vi "Convert a number to its letter.vi"(2 "Number":i32, 3 "ordered item type (default)":T1(ring)) -> (1 "string":string)   [LabVIEW 2015, in "NI_ReportGenerationCore.lvlib"]
uses:
  <vilib>/Utility/NIReport.llb/NI_ReportGenerationCore.lvlib
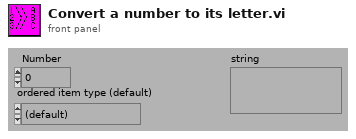
[diagram p1: front panel]
types:
  T1 = enum16{"(default)", "arabic numerals", "lower alpha", "upper alpha"}
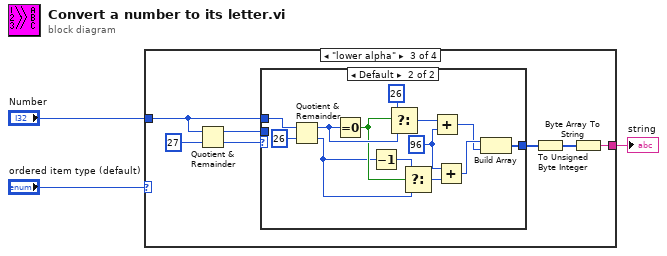
[diagram p0: block diagram]
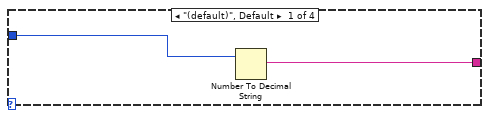
[diagram p2: hidden frame]
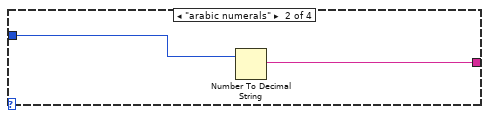
[diagram p3: hidden frame]
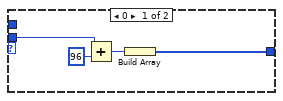
[diagram p4: hidden frame]
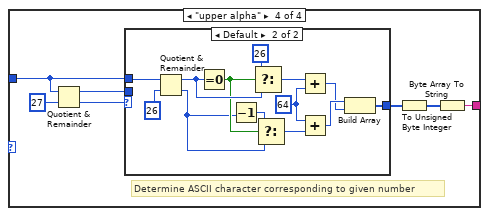
[diagram p5: hidden frame]
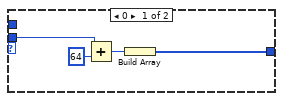
[diagram p6: hidden frame]
diagram:
  n1 = case shown="\"lower alpha\"" "ordered item type (default)" {
    tunnel: [w5 w7 w10 w34] -> w3
    tunnel: "Number" -> [w4 w6 w9 w33]
    frame "(default)", Default {
      n2 = Number To Decimal String(number=w4) -> (decimal integer string=w5:string)  [unwired: 1 out]
    }
    frame "arabic numerals" {
      n3 = Number To Decimal String(number=w6) -> (decimal integer string=w7:string)  [unwired: 1 out]
    }
    frame "lower alpha" {
      n4 = Quotient & Remainder(x=w9, y=27) -> (x-y*floor(x/y)=w13:i32, floor(x/y)=w8:i32)
      n5 = case shown="Default" w8 {
        tunnel: w9 -> [_ w19]
        tunnel: w13 -> [w18 _]
        tunnel: [w17 w21] -> w12
        frame 0 {
          n6 = Add(x=w18, y=96) -> (x+y=w15:i32)
          n7 = Build Array(w15) -> (w17:i32[])
        }
        frame Default {
          w20 = 96
          n8 = Quotient & Remainder(x=w19, y=26) -> (x-y*floor(x/y)=w29:i32, floor(x/y)=w26:i32)
          n9 = Equal To 0?(x=w29) -> (x = 0?=w27:bool)
          n10 = Decrement(x=w26) -> (x-1=w28:i32)
          n11 = Select(t=26, s=w27, f=w29) -> (s? t:f=w25:i32)
          n12 = Select(t=w28, s=w27, f=w26) -> (s? t:f=w24:i32)
          n13 = Add(x=w25, y=w20) -> (x+y=w22:i32)
          n14 = Add(x=w20, y=w24) -> (x+y=w23:i32)
          n15 = Build Array(w23, w22) -> (w21:i32[])
        }
      }
      n16 = To Unsigned Byte Integer(number=w12) -> (unsigned 8bit integer=w11:u8[])
      n17 = Byte Array To String(unsigned byte array=w11) -> (string=w10:string)
    }
    frame "upper alpha" {
      # "Determine ASCII character corresponding to given number"
      n18 = Quotient & Remainder(x=w33, y=27) -> (x-y*floor(x/y)=w37:i32, floor(x/y)=w32:i32)
      n19 = case shown="Default" w32 {
        tunnel: w33 -> [_ w43]
        tunnel: w37 -> [w42 _]
        tunnel: [w41 w45] -> w36
        frame 0 {
          n20 = Add(x=w42, y=64) -> (x+y=w39:i32)
          n21 = Build Array(w39) -> (w41:i32[])
        }
        frame Default {
          w44 = 64
          n22 = Quotient & Remainder(x=w43, y=26) -> (x-y*floor(x/y)=w53:i32, floor(x/y)=w50:i32)
          n23 = Equal To 0?(x=w53) -> (x = 0?=w51:bool)
          n24 = Decrement(x=w50) -> (x-1=w52:i32)
          n25 = Select(t=26, s=w51, f=w53) -> (s? t:f=w49:i32)
          n26 = Select(t=w52, s=w51, f=w50) -> (s? t:f=w48:i32)
          n27 = Add(x=w49, y=w44) -> (x+y=w46:i32)
          n28 = Add(x=w44, y=w48) -> (x+y=w47:i32)
          n29 = Build Array(w47, w46) -> (w45:i32[])
        }
      }
      n30 = To Unsigned Byte Integer(number=w36) -> (unsigned 8bit integer=w35:u8[])
      n31 = Byte Array To String(unsigned byte array=w35) -> (string=w34:string)
    }
  }
  "string" <- w3
